vi "Sort Complex Numbers.vi"(9 "method":u16(ring) items=["Real, Imaginary", "Magnitude, Real, Imaginary", "Magnitude, Phase Angle"], 10 "order":enum16{"Ascending", "Descending"}(ring), 11 "Complex Numbers":cdb[](array[numeric]) format="%#.6g") -> (0 "error":i32, 2 "Sorted Index":i32[](array[numeric]), 3 "Sorted Complex Numbers":cdb[](array[numeric]) format="%#.6g")   [LabVIEW 2020, in "NI_AALPro.lvlib"]
doc: "Sorts an array of complex numbers in ascending or descending order with respect to real and imaginary parts or magnitude."
uses:
  <vilib>/Analysis/NI_AALPro.lvlib
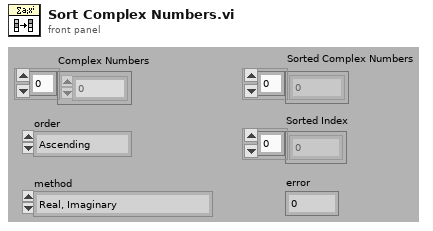
[diagram p1: front panel]
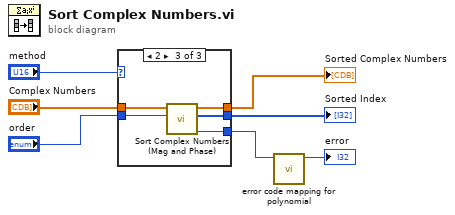
[diagram p0: block diagram]
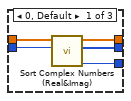
[diagram p2: hidden frame]
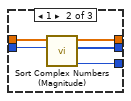
[diagram p3: hidden frame]
diagram:
  n1 = case shown="2" "method" {
    tunnel: "Complex Numbers" -> [w12 w17 w22]
    tunnel: "order" -> [w11 w16 w21]
    tunnel: [w10 w15 w20] -> w4
    tunnel: [w9 w14 w19] -> w3
    tunnel: [w8 w13 w18] -> w2
    frame 0, Default {
      n2 = call <vilib>:"Sort Complex Numbers (Real&Imag).vi"("Order"=w11, "Complex Numbers"=w12) -> ("error"=w8:i32, "Sorted Index"=w9:i32[], "Sorted Complex Numbers"=w10:cdb[])  [unwired: 7 in]
    }
    frame 1 {
      n3 = call <vilib>:"Sort Complex Numbers (Magnitude).vi"("Order"=w16, "Complex Numbers"=w17) -> ("error"=w13:i32, "Sorted Index"=w14:i32[], "Sorted Complex Numbers"=w15:cdb[])  [unwired: 7 in]
    }
    frame 2 {
      n4 = call <vilib>:"Sort Complex Numbers (Mag and Phase).vi"("Order"=w21, "Complex Numbers"=w22) -> ("error"=w18:i32, "Sorted Index"=w19:i32[], "Sorted Complex Numbers"=w20:cdb[])  [unwired: 7 in]
    }
  }
  "Sorted Complex Numbers" <- w4
  "Sorted Index" <- w3
  n5 = call <vilib>:"error code mapping for polynomial.vi"("error in"=w2) -> ("error out"=→"error":i32)  [unwired: 10 in]
